vi "4Pi Drift Monitor.vi"() -> ()   [LabVIEW 2021]
uses:
  <vilib>/vision/Image Controls.llb/IMAQ Image.ctl
  4Pi Drift Monitor Controls/4Pi Drift Monitor - Notifier Type.ctl
  4Pi Drift Monitor Controls/4Pi Drift Monitor - Actions.ctl
  Hardware Configuration/Hardware Configuration Controls/Device Type.ctl
  Hardware Configuration/Hardware Configuration Controls/Device Function.ctl
panel:
  in  "CCD Offset":dbl=100.0
  in  "Offset Position Scale":dbl=2.0
  out "ROI Stack":u16[][][](array[numeric])
  out "Y (nm)":cluster{dbl, dbl, dbl, dbl}(graph)
  in  "Quit":bool
  out "Init X pos (px)":dbl[](array[numeric])
  out "Init Y pos (px)":dbl[](array[numeric])
  out "Y pos (px)":dbl[](array[numeric])
  out "X pos (px)":dbl[](array[numeric])
  in  "Frame Accumulation":i32
  in  "ROI Size":i32=7
  in  "Camera Px. Size (nm)":dbl=0.1
  in  "qd4":bool=TRUE
  in  "qd3":bool=TRUE
  in  "qd2":bool=TRUE
  in  "qd1":bool=TRUE
  out "X (nm)":cluster{dbl, dbl, dbl, dbl}(graph)
  in  "Start Monitor":bool
  # "Quadrant"
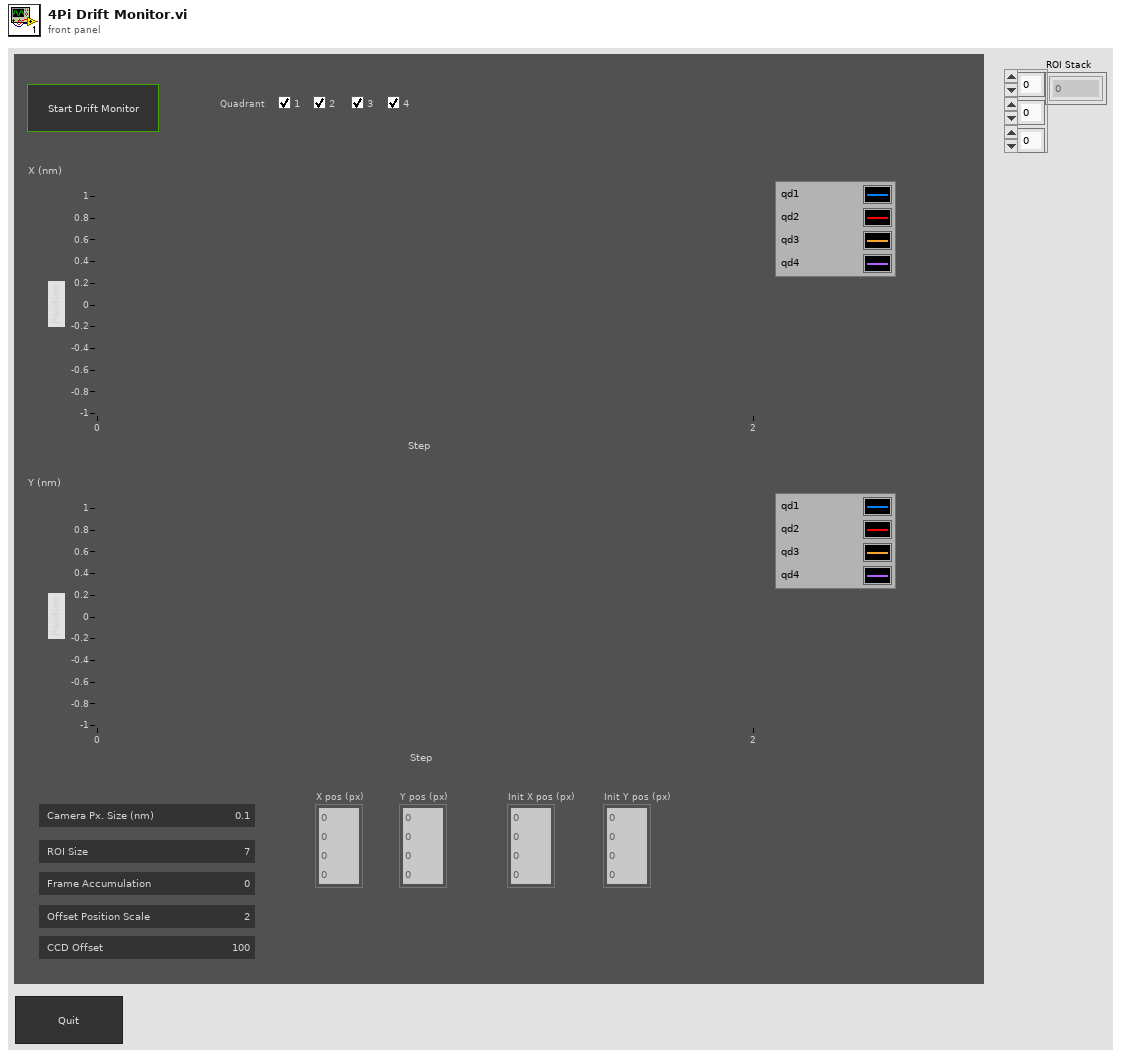
[diagram p1: front panel]
types:
  T1 = typedef "4Pi Drift Monitor - Actions.ctl" = enum16{"Idle", "Start Monitor", "Get Initial XY Pos", "Get Initial Image", "Get Image", "Get XY Position", "Update Plots", "Exit Loop", "Abort", "Quit"}
  T2 = typedef "4Pi Drift Monitor - Notifier Type.ctl" = cluster{"Action":T1, "Frame Accums.":u16, "Camera Px. Size (nm)":dbl, "QD On/Off":bool[], "Image Ref":T3[], "ROI Size":i32, "Frame Accumulation":u16, "ROI Stack":u16[][][], "Running?":bool}
  T3 = typedef "IMAQ Image.ctl" = refnum<image>
  T4 = typedef "Device Function.ctl" = enum16{"Primary", "Secondary", "Overview", "Wide Field Drift Correction", "642 nm Excitation", "560 nm Excitation", "940 nm Excitation", "546 nm Excitation", "488 nm Excitation", "405 nm Excitation", "Objective Drift Correction", "4Pi Focus Lock", "4Pi Objective Lock", "Objective XY", "Objective Z", "Sample XY", "Sample Coarse Z", "Sample Z", "4Pi Lower", "4Pi Upper", "Em Small", "Em Large", "Ex Small", "Ex Large", "Mojo", "Adj Cavity", "Line Scanning", "Alert"}
  T5 = typedef "Device Type.ctl" = enum16{"AOTF", "Camera", "Deformable Mirror", "Laser", "Flip Mirror", "Shutter", "Stage", "Waveform", "FPGA", "Email"}
  T6 = typedef "4Pi OBJ Lock-2D Gaussian - Best Fit Parameters.ctl" = cluster{"Amplitude":dbl, "X Position":dbl, "Y Position":dbl, "X Width":dbl, "Y Width":dbl, "Offset":dbl}
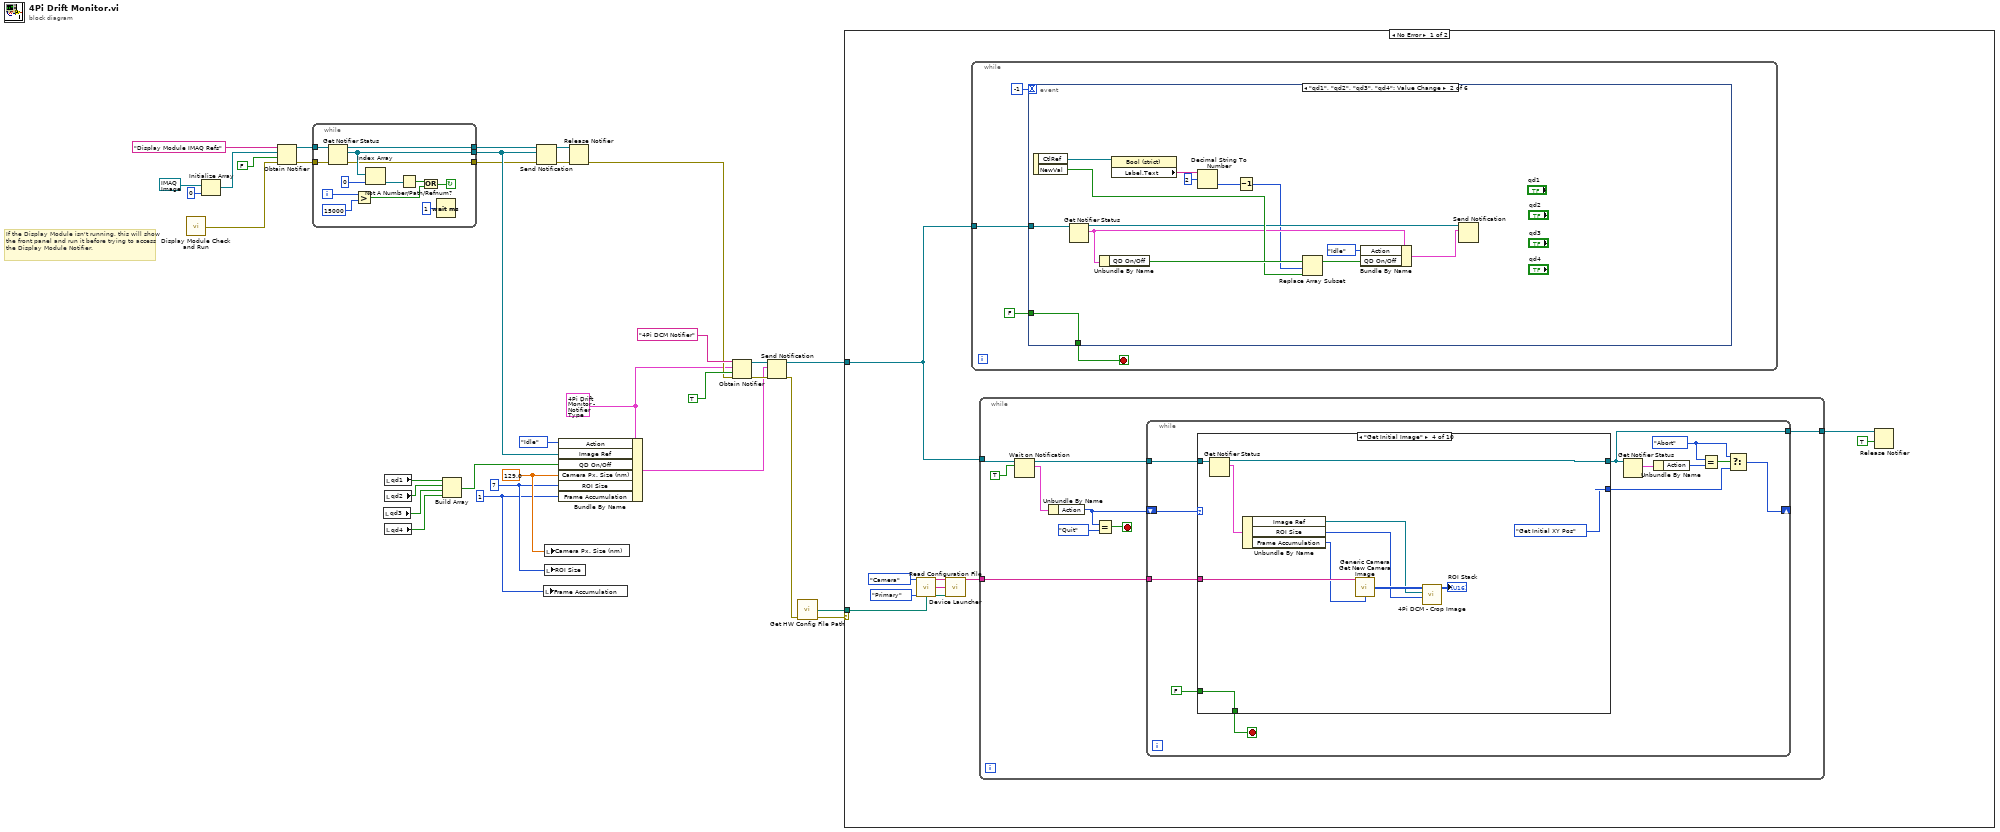
[diagram p0: block diagram]
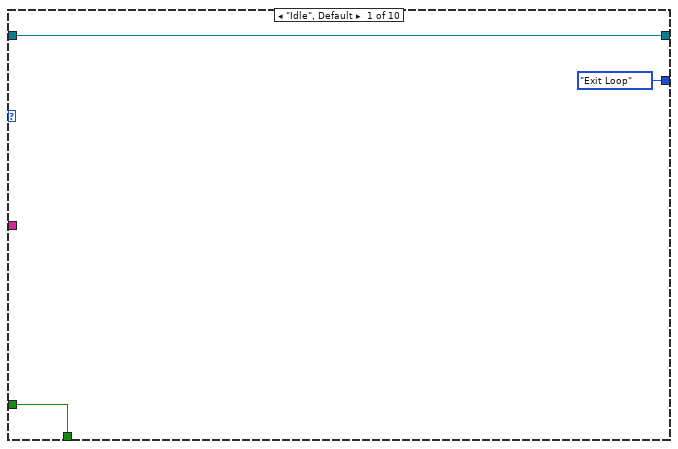
[diagram p2: hidden frame]
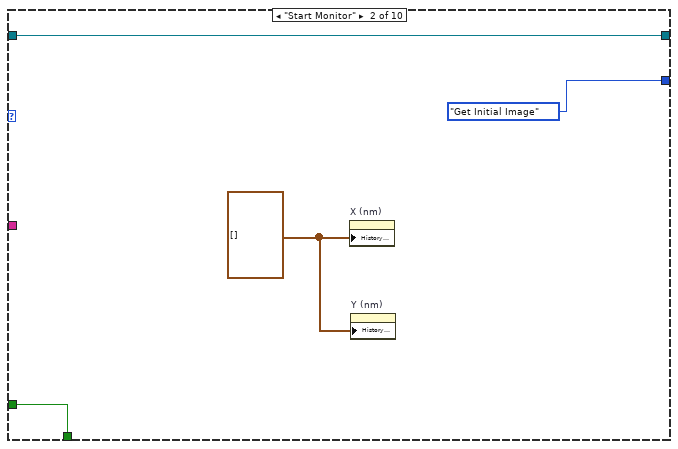
[diagram p3: hidden frame]
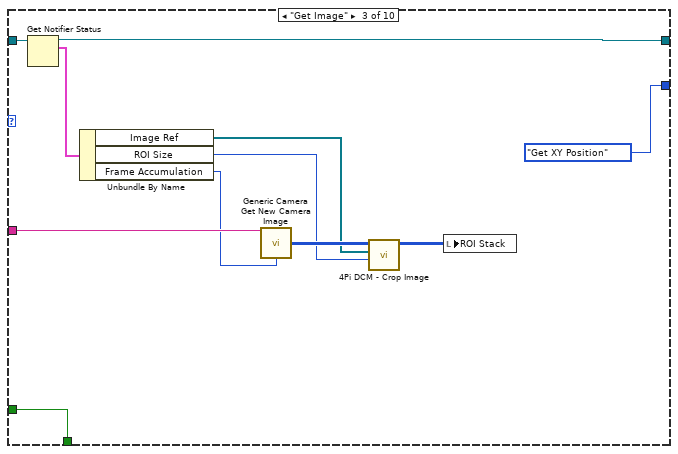
[diagram p4: hidden frame]
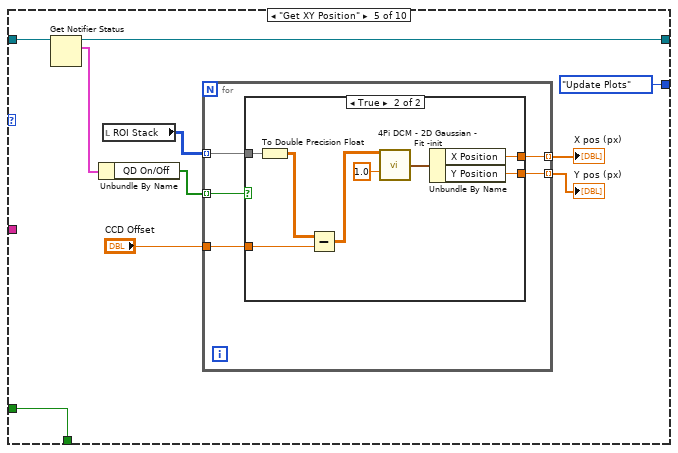
[diagram p5: hidden frame]
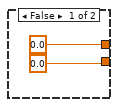
[diagram p6: hidden frame]
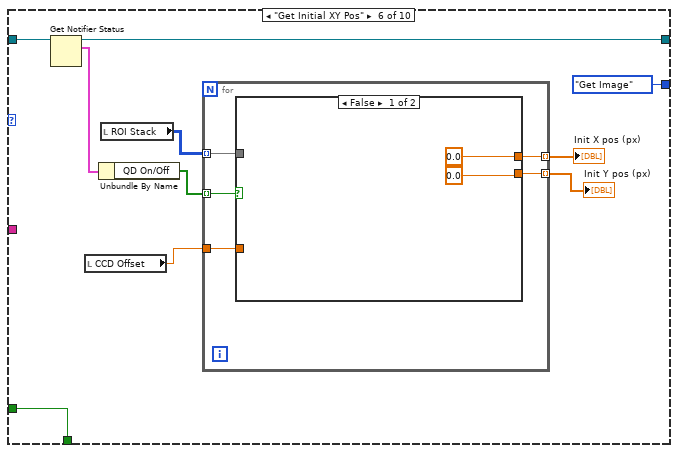
[diagram p7: hidden frame]
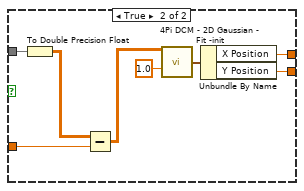
[diagram p8: hidden frame]
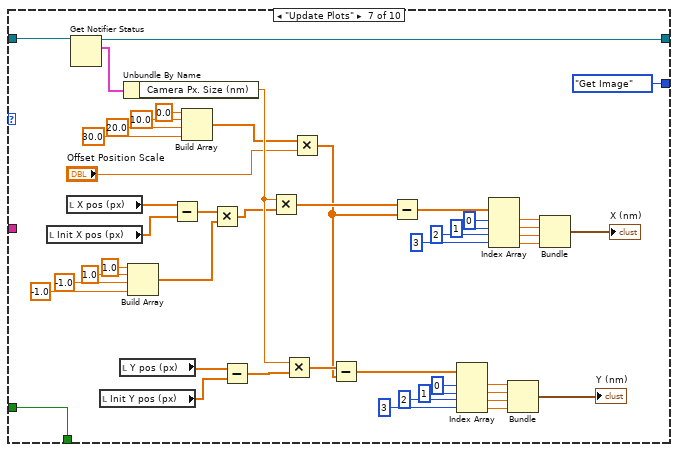
[diagram p9: hidden frame]
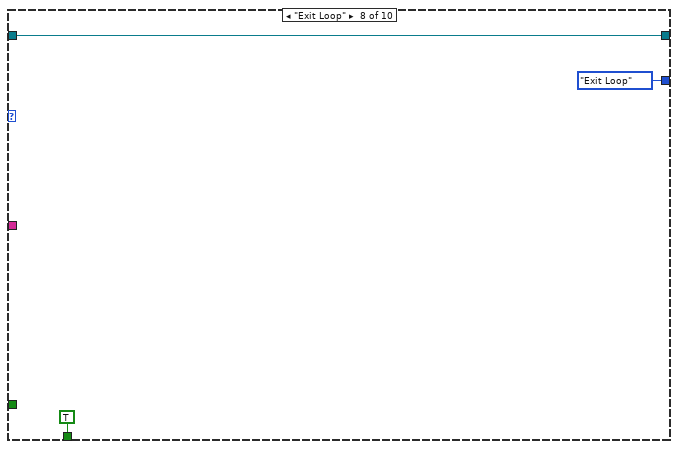
[diagram p10: hidden frame]
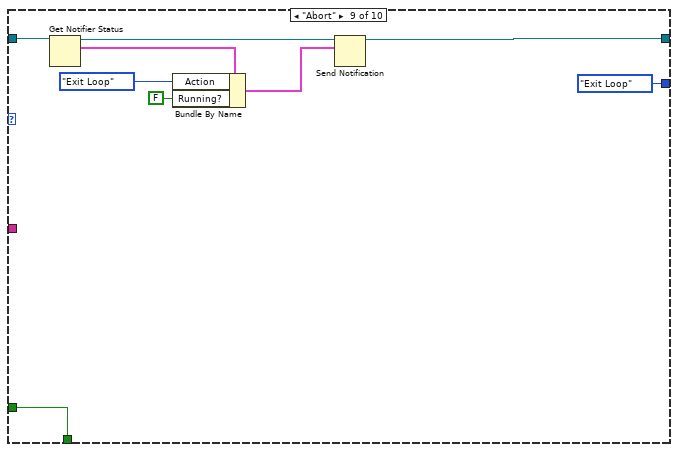
[diagram p11: hidden frame]
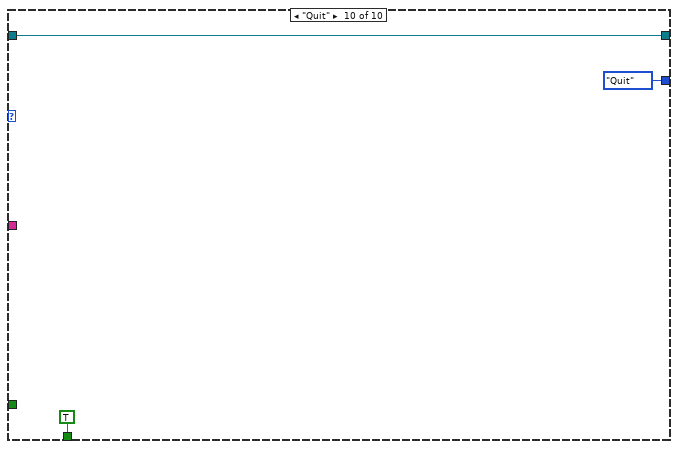
[diagram p12: hidden frame]
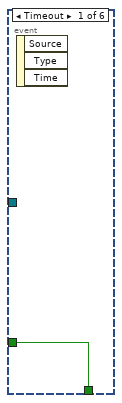
[diagram p13: hidden frame]
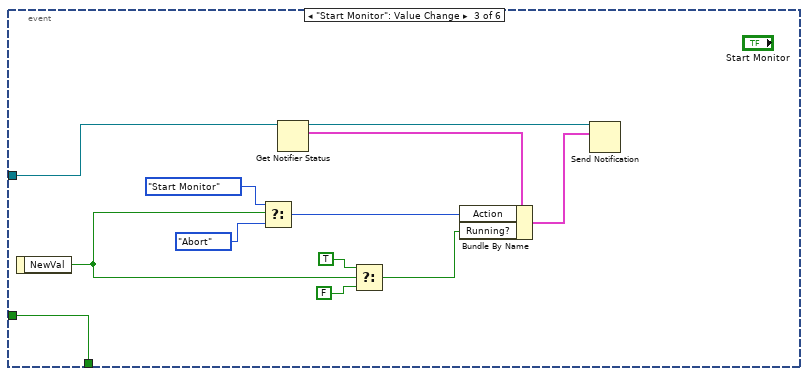
[diagram p14: hidden frame]
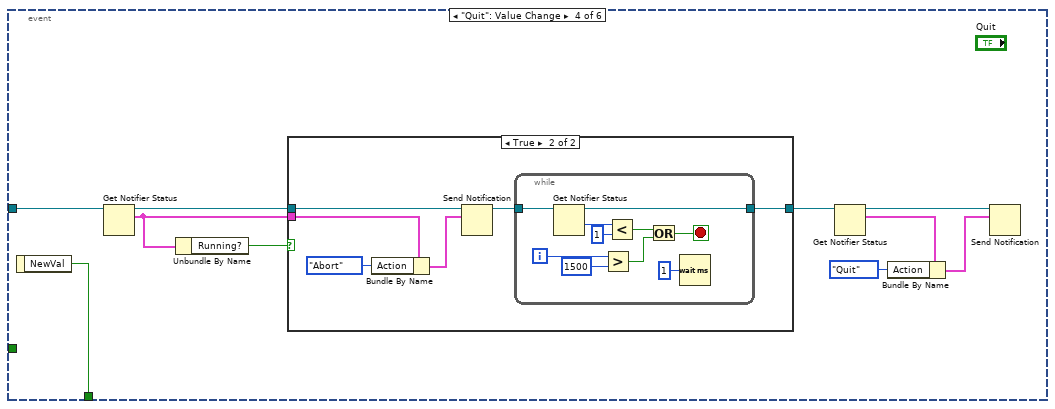
[diagram p15: hidden frame]
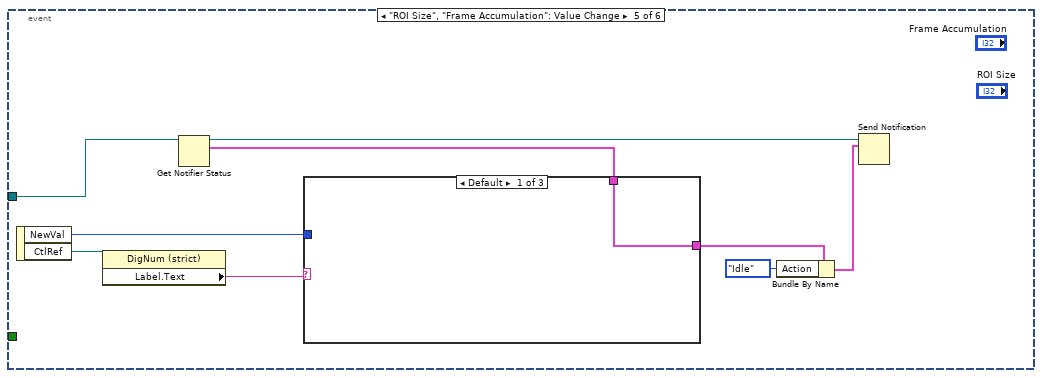
[diagram p17: hidden frame]
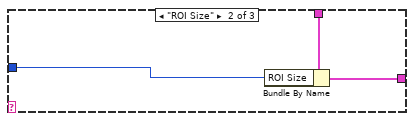
[diagram p18: hidden frame]
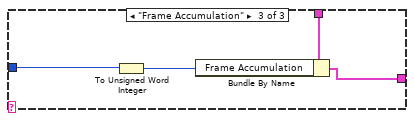
[diagram p19: hidden frame]
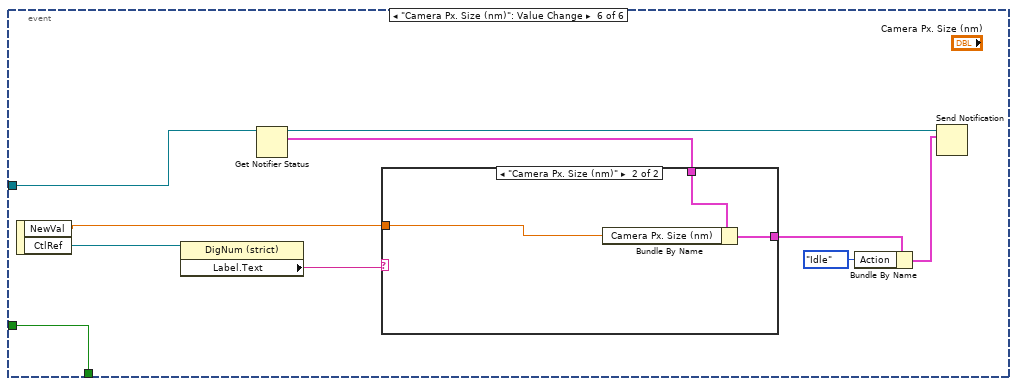
[diagram p20: hidden frame]
diagram:
  w2 = u16 1 ("Frame Accumulation")
  w3 = 7 ("ROI Size")
  w4 = 129.0 ("Camera Px. Size (nm)")
  w1 = T2 {"Action"=enum."Start Monitor", "Frame Accums."=0, "Camera Px. Size (nm)"=0.1, "QD On/Off"=[], "Image Ref"=[], "ROI Size"=0, "Frame Accumulation"=0, "ROI Stack"=[], "Running?"=FALSE} ("4Pi Drift Monitor Notifier Type")
  # "If the Display Module isn't running, this will show the front panel and run it before trying to access the Display Module Notifier."
  n1 = call "Display Module Check and Run.vi"() -> ("Error"=w29:errorcluster)  [unwired: 15 in]
  n2 = Initialize Array(T3 refnum ("New Image"), 0 ("dimension size")) -> (w26:T3[])
  n3 = Obtain Notifier(name (unnamed)="Display Module IMAQ Refs", notification data type=w26, create if not found? (T)=FALSE, error in (no error)=w29) -> (notifier out=w28:refnum<notifier>, error out=w27:errorcluster)  [unwired: 1 out]
  n4 = while {
    tunnel: w28 -> [w46]
    tunnel: w27 -> [w45]
    tunnel: [w44] -> w8
    tunnel: [w43] -> w7
    tunnel: [w39] -> w6
    i -> [w38]
    stop <- w35 continue-if-true
    n5 = Get Notifier Status(notifier=w46, error in (no error)=w45) -> (notifier out=w44:refnum<notifier>, current notification=w43:T3[], error out=w39:errorcluster)  [unwired: 2 out]
    n6 = Greater?(x=w38, y=15000) -> (0:w34:bool)
    n7 = Index Array(array=w43, index=0) -> (element=w41:T3)
    n8 = Not A Number/Path/Refnum?(number/path/refnum=w41) -> (NaN/Path/Refnum?=w36:bool)
    n9 = Or(x=w36, y=w34) -> (x .or. y?=w35:bool)
    n10 = Wait (ms)(milliseconds to wait=u32 1) -> ()  [unwired: 1 out]
  }
  n11 = local read "qd3"() -> (w13:bool)
  n12 = local read "qd1"() -> (w15:bool)
  n13 = local read "qd2"() -> (w14:bool)
  n14 = local read "qd4"() -> (w12:bool)
  n15 = Build Array(w15, w14, w13, w12) -> (w11:bool[])
  n16 = Send Notification(notification=w7, notifier=w8, error in (no error)=w6) -> (notifier out=w9:refnum<notifier>, error out=w10:errorcluster)
  n17 = local write "Frame Accumulation"(w2) -> ()
  n18 = local write "Camera Px. Size (nm)"(w4) -> ()
  n19 = local write "ROI Size"(w3) -> ()
  n20 = Bundle By Name(cluster=w1, "Action"=4Pi_Drift_Monitor_-_Actions."Idle", "Image Ref"=w7, "QD On/Off"=w11, "Camera Px. Size (nm)"=w4, "ROI Size"=w3, "Frame Accumulation"=w2) -> (w17:T2)
  n21 = Release Notifier(notifier=w9, error in (no error)=w10) -> (error out=w5:errorcluster)  [unwired: 1 in, 2 out]
  n22 = Obtain Notifier(name (unnamed)="4Pi DCM Notifier", notification data type=w1, create if not found? (T)=TRUE, error in (no error)=w5) -> (notifier out=w24:refnum<notifier>, error out=w22:errorcluster)  [unwired: 1 out]
  n23 = Send Notification(notification=w17, notifier=w24, error in (no error)=w22) -> (notifier out=w16:refnum<notifier>, error out=w21:errorcluster)
  n24 = call "Get HW Config File Path.vi"("Error"=w21) -> ("File Path"=w19:path, "Error"=w20:errorcluster)  [unwired: 13 in]
  n25 = case shown="No Error" w20 {
    tunnel: w19 -> [w53 _]
    tunnel: w16 -> [w49 _]
    frame No Error {
      n26 = call "Read Configuration File.vi"("Device Type"=Device_Type."Camera", "Device Function"=Device_Function."Primary", "Config File Path"=w53) -> ("Unique Notifier Name"=w54:string, "Device Ports/IDs/Channels"=w56:string[], "Device Engine Path"=w55:path)  [unwired: 9 in, 1 out]
      n27 = call "Device Launcher.vi"("Notifier Name"=w54, "Device Ports/IDs/Channels"=w56, "Device Engine Path"=w55) -> ("Notifier Name"=w50:string)  [unwired: 11 in, 1 out]
      n28 = while {
        tunnel: w49 -> [w222]
        stop <- w221 stop-if-true
        n29 = event shown="[1] \"qd1\", \"qd2\", \"qd3\", \"qd4\": Value Change" {
          selector: _ -> [_ _ _ _ _ _]
          dyn-events: _ -> [_ _ _ _ _ _]
          timeout: -1 -> [_ _ _ _ _ _]
          tunnel: w222 -> [_ w236 w240 w251 w283 w294]
          tunnel: [w223 w226 w243 w259 _ w303] -> w221
          tunnel: FALSE -> [w223 w226 w243 _ _ w303]
          event Timeout {
            n30 = event-data() -> ()  [unwired: 1 in, 3 out]
          }
          event "qd1", "qd2", "qd3", "qd4": Value Change {
            n31 = event-data() -> ("CtlRef"=w237:refnum<vi>, "NewVal"=w232:bool)  [unwired: 1 in]
            n32 = Get Notifier Status(notifier=w236) -> (notifier out=w228:refnum<notifier>, current notification=w231:T2)  [unwired: 1 in, 3 out]
            n33 = Unbundle By Name(w231) -> ("QD On/Off"=w235:bool[])
            n34 = property class="Bool (strict)"(reference=w237) -> ("Label.Text"=w234:string)  [unwired: 1 in, 2 out]
            n35 = Decimal String To Number(string=w234, offset=2 ("offset (0)")) -> (number=w225:i32)  [unwired: 1 in, 1 out]
            n36 = Decrement(x=w225) -> (x-1=w224:i32)
            n37 = Replace Array Subset(array=w235, new element=w232, index=w224) -> (w230:bool[])
            n38 = Bundle By Name(cluster=w231, "Action"=4Pi_Drift_Monitor_-_Actions."Idle", "QD On/Off"=w230) -> (w229:T2)
            n39 = Send Notification(notification=w229, notifier=w228) -> ()  [unwired: 1 in, 2 out]
          }
          event "Start Monitor": Value Change {
            n40 = event-data() -> ("NewVal"=w239:bool)  [unwired: 1 in]
            n41 = Select(t=4Pi_Drift_Monitor_-_Actions."Start Monitor" ("Action"), s=w239, f=4Pi_Drift_Monitor_-_Actions."Abort") -> (s? t:f=w246:T1)
            n42 = Get Notifier Status(notifier=w240) -> (notifier out=w244:refnum<notifier>, current notification=w249:T2)  [unwired: 1 in, 3 out]
            n43 = Select(t=TRUE ("Running?"), s=w239, f=FALSE) -> (s? t:f=w238:bool)
            n44 = Bundle By Name(cluster=w249, "Action"=w246, "Running?"=w238) -> (w245:T2)
            n45 = Send Notification(notification=w245, notifier=w244) -> ()  [unwired: 1 in, 2 out]
          }
          event "Quit": Value Change {
            n46 = event-data() -> ("NewVal"=w259:bool)  [unwired: 1 in]
            n47 = Get Notifier Status(notifier=w251) -> (notifier out=w254:refnum<notifier>, current notification=w252:T2)  [unwired: 1 in, 3 out]
            n48 = Unbundle By Name(w252) -> ("Running?"=w255:bool)
            n49 = case shown="True" w255 {
              tunnel: w254 -> [w260 w265]
              tunnel: [w260 w262] -> w253
              tunnel: w252 -> [_ w266]
              frame False {
              }
              frame True {
                n50 = Bundle By Name(cluster=w266, "Action"=4Pi_Drift_Monitor_-_Actions."Abort") -> (w264:T2)
                n51 = Send Notification(notification=w264, notifier=w265) -> (notifier out=w263:refnum<notifier>)  [unwired: 1 in, 1 out]
                n52 = while {
                  tunnel: w263 -> [w276]
                  tunnel: [w271] -> w262
                  i -> [w270]
                  stop <- w272 stop-if-true
                  n53 = Get Notifier Status(notifier=w276) -> (notifier out=w271:refnum<notifier>, # waiting=w275:i32)  [unwired: 1 in, 3 out]
                  n54 = Greater?(x=w270, y=1500) -> (0:w268:bool)
                  n55 = Less?(x=w275, y=1) -> (x < y?=w273:bool)
                  n56 = Or(x=w273, y=w268) -> (x .or. y?=w272:bool)
                  n57 = Wait (ms)(milliseconds to wait=u32 1) -> ()  [unwired: 1 out]
                }
              }
            }
            n58 = Get Notifier Status(notifier=w253) -> (notifier out=w257:refnum<notifier>, current notification=w258:T2)  [unwired: 1 in, 3 out]
            n59 = Bundle By Name(cluster=w258, "Action"=4Pi_Drift_Monitor_-_Actions."Quit") -> (w256:T2)
            n60 = Send Notification(notification=w256, notifier=w257) -> ()  [unwired: 1 in, 2 out]
          }
          event "ROI Size", "Frame Accumulation": Value Change {
            n61 = event-data() -> ("NewVal"=w281:i32, "CtlRef"=w285:refnum<vi>)  [unwired: 1 in]
            n62 = property class="DigNum (strict)"(reference=w285) -> ("Label.Text"=w284:string)  [unwired: 1 in, 2 out]
            n63 = Get Notifier Status(notifier=w283) -> (notifier out=w280:refnum<notifier>, current notification=w282:T2)  [unwired: 1 in, 3 out]
            n64 = case shown="Default" w284 {
              tunnel: w282 -> [w286 w289 w293]
              tunnel: w281 -> [_ w288 w291]
              tunnel: [w286 w287 w292] -> w279
              frame Default {
              }
              frame "ROI Size" {
                n65 = Bundle By Name(cluster=w289, "ROI Size"=w288) -> (w287:T2)
              }
              frame "Frame Accumulation" {
                n66 = To Unsigned Word Integer(number=w291) -> (unsigned 16bit integer=w290:u16)
                n67 = Bundle By Name(cluster=w293, "Frame Accumulation"=w290) -> (w292:T2)
              }
            }
            n68 = Bundle By Name(cluster=w279, "Action"=4Pi_Drift_Monitor_-_Actions."Idle") -> (w277:T2)
            n69 = Send Notification(notification=w277, notifier=w280) -> ()  [unwired: 1 in, 2 out]
          }
          event "Camera Px. Size (nm)": Value Change {
            n70 = event-data() -> ("NewVal"=w295:dbl, "CtlRef"=w296:refnum<vi>)  [unwired: 1 in]
            n71 = property class="DigNum (strict)"(reference=w296) -> ("Label.Text"=w302:string)  [unwired: 1 in, 2 out]
            n72 = Get Notifier Status(notifier=w294) -> (notifier out=w300:refnum<notifier>, current notification=w301:T2)  [unwired: 1 in, 3 out]
            n73 = case shown="\"Camera Px. Size (nm)\"" w302 {
              tunnel: w301 -> [w304 w307]
              tunnel: w295 -> [_ w306]
              tunnel: [w304 w305] -> w299
              frame Default {
              }
              frame "Camera Px. Size (nm)" {
                n74 = Bundle By Name(cluster=w307, "Camera Px. Size (nm)"=w306) -> (w305:T2)
              }
            }
            n75 = Bundle By Name(cluster=w299, "Action"=4Pi_Drift_Monitor_-_Actions."Idle") -> (w297:T2)
            n76 = Send Notification(notification=w297, notifier=w300) -> ()  [unwired: 1 in, 2 out]
          }
        }
      }
      n77 = while {
        tunnel: w50 -> [w59]
        tunnel: w49 -> [w63]
        tunnel: [w57] -> w47
        stop <- w61 stop-if-true
        n78 = Wait on Notification(notifier=w63, ignore previous (F)=TRUE) -> (notifier out=w60:refnum<notifier>, notification=w64:T2)  [unwired: 2 in, 2 out]
        n79 = Unbundle By Name(w64) -> ("Action"=w58:T1)
        n80 = Equal?(x=w58, y=4Pi_Drift_Monitor_-_Actions."Quit") -> (x = y?=w61:bool)
        n81 = while {
          tunnel: w60 -> [w77]
          tunnel: w59 -> [w76]
          shift-right: [w70] -> _
          shift-left: w58 -> [w69]
          tunnel: [w66] -> w57
          stop <- w68 stop-if-true
          w72 = 4Pi_Drift_Monitor_-_Actions."Abort" ("x")
          n82 = case shown="\"Get Initial Image\"" w69 {
            tunnel: [w79 w84 w86 w97 w111 w136 w177 w206 w209 w216] -> w66
            tunnel: w77 -> [w79 w84 w95 w106 w116 w141 w203 w206 w215 w216]
            tunnel: w76 -> [_ _ w94 w105 _ _ _ _ _ _]
            tunnel: [4Pi_Drift_Monitor_-_Actions."Exit Loop" ("y") 4Pi_Drift_Monitor_-_Actions."Get Initial Image" ("y") 4Pi_Drift_Monitor_-_Actions."Get XY Position" ("y") 4Pi_Drift_Monitor_-_Actions."Get Initial XY Pos" ("y") 4Pi_Drift_Monitor_-_Actions."Update Plots" ("y") 4Pi_Drift_Monitor_-_Actions."Get Image" ("y") 4Pi_Drift_Monitor_-_Actions."Get Image" ("y") 4Pi_Drift_Monitor_-_Actions."Exit Loop" ("y") 4Pi_Drift_Monitor_-_Actions."Exit Loop" ("y") 4Pi_Drift_Monitor_-_Actions."Quit" ("y")] -> w71
            tunnel: [w78 w81 w87 w98 w110 w135 w176 TRUE w208 TRUE] -> w68
            tunnel: FALSE -> [w78 w81 w87 w98 w110 w135 w176 _ w208 _]
            frame "Idle", Default {
            }
            frame "Start Monitor" {
              w82 = cluster{dbl, dbl, dbl, dbl}[] [] ("History Data")
              n83 = property on="X (nm)" class="WFChart (strict)"("History Data"=w82) -> ()  [unwired: 2 in, 2 out]
              n84 = property on="Y (nm)" class="WFChart (strict)"("History Data"=w82) -> ()  [unwired: 2 in, 2 out]
            }
            frame "Get Image" {
              n85 = Get Notifier Status(notifier=w95) -> (notifier out=w86:refnum<notifier>, current notification=w89:T2)  [unwired: 1 in, 3 out]
              n86 = Unbundle By Name(w89) -> ("Image Ref"=w92:T3[], "ROI Size"=w91:i32, "Frame Accumulation"=w90:u16)
              n87 = call "Generic Camera Get New Camera Image.vi"("Camera Notifier Name"=w94, "Frames"=w90) -> ("Image - U16"=w93:u16[][])  [unwired: 11 in, 2 out]
              n88 = call "4Pi DCM - Crop Image.vi"("ROI Size"=w91, "Image Refs"=w92, "Input Image (U16)"=w93) -> ("Output Image Stack"=w85:u16[][][])  [unwired: 8 in]
              n89 = local write "ROI Stack"(w85) -> ()
            }
            frame "Get Initial Image" {
              n90 = Get Notifier Status(notifier=w106) -> (notifier out=w97:refnum<notifier>, current notification=w100:T2)  [unwired: 1 in, 3 out]
              n91 = Unbundle By Name(w100) -> ("Image Ref"=w103:T3[], "ROI Size"=w102:i32, "Frame Accumulation"=w101:u16)
              n92 = call "Generic Camera Get New Camera Image.vi"("Camera Notifier Name"=w105, "Frames"=w101) -> ("Image - U16"=w104:u16[][])  [unwired: 11 in, 2 out]
              n93 = call "4Pi DCM - Crop Image.vi"("ROI Size"=w102, "Image Refs"=w103, "Input Image (U16)"=w104) -> ("Output Image Stack"=→"ROI Stack":u16[][][])  [unwired: 8 in]
            }
            frame "Get XY Position" {
              n94 = Get Notifier Status(notifier=w116) -> (notifier out=w111:refnum<notifier>, current notification=w115:T2)  [unwired: 1 in, 3 out]
              n95 = Unbundle By Name(w115) -> ("QD On/Off"=w109:bool[])
              n96 = local read "ROI Stack"() -> (w108:u16[][][])
              n97 = for {
                tunnel: w108 -> [w121] mode=indexing
                tunnel: [w120] -> w114 mode=indexing
                tunnel: [w119] -> w113 mode=indexing
                tunnel: w109 -> [w118] mode=indexing
                tunnel: "CCD Offset" -> [w117]
                n98 = case shown="True" w118 {
                  tunnel: w121 -> [_ w131]
                  tunnel: [0.0 ("X Position") w128] -> w120
                  tunnel: [0.0 ("Y Position") w127] -> w119
                  tunnel: w117 -> [_ w125]
                  frame False {
                  }
                  frame True {
                    n99 = To Double Precision Float(number=w131) -> (double precision float=w126:dbl[][])
                    n100 = Subtract(x=w126, y=w125) -> (x-y=w124:dbl[][])
                    n101 = call "4Pi DCM - 2D Gaussian - Fit -init.vi"("Image In (DBL)"=w124, "width"=1.0) -> ("Best Fit Params"=w129:T6)  [unwired: 12 in, 1 out]
                    n102 = Unbundle By Name(w129) -> ("X Position"=w128:dbl, "Y Position"=w127:dbl)
                  }
                }
              }
              "X pos (px)" <- w114
              "Y pos (px)" <- w113
            }
            frame "Get Initial XY Pos" {
              n103 = Get Notifier Status(notifier=w141) -> (notifier out=w136:refnum<notifier>, current notification=w140:T2)  [unwired: 1 in, 3 out]
              n104 = local read "CCD Offset"() -> (w132:dbl)
              n105 = Unbundle By Name(w140) -> ("QD On/Off"=w134:bool[])
              n106 = local read "ROI Stack"() -> (w133:u16[][][])
              n107 = for {
                tunnel: w133 -> [w146] mode=indexing
                tunnel: [w145] -> w139 mode=indexing
                tunnel: [w144] -> w138 mode=indexing
                tunnel: w134 -> [w143] mode=indexing
                tunnel: w132 -> [w142]
                n108 = case shown="False" w143 {
                  tunnel: w146 -> [_ w156]
                  tunnel: [0.0 ("X Position") w153] -> w145
                  tunnel: [0.0 ("Y Position") w152] -> w144
                  tunnel: w142 -> [_ w150]
                  frame False {
                  }
                  frame True {
                    n109 = To Double Precision Float(number=w156) -> (double precision float=w151:dbl[][])
                    n110 = Subtract(x=w151, y=w150) -> (x-y=w149:dbl[][])
                    n111 = call "4Pi DCM - 2D Gaussian - Fit -init.vi"("Image In (DBL)"=w149, "width"=1.0) -> ("Best Fit Params"=w154:T6)  [unwired: 12 in, 1 out]
                    n112 = Unbundle By Name(w154) -> ("X Position"=w153:dbl, "Y Position"=w152:dbl)
                  }
                }
              }
              "Init X pos (px)" <- w139
              "Init Y pos (px)" <- w138
            }
            frame "Update Plots" {
              n113 = local read "Init X pos (px)"() -> (w200:dbl[])
              n114 = local read "X pos (px)"() -> (w201:dbl[])
              n115 = Get Notifier Status(notifier=w203) -> (notifier out=w177:refnum<notifier>, current notification=w202:T2)  [unwired: 1 in, 3 out]
              n116 = local read "Init Y pos (px)"() -> (w197:dbl[])
              n117 = local read "Y pos (px)"() -> (w198:dbl[])
              n118 = Unbundle By Name(w202) -> ("Camera Px. Size (nm)"=w196:dbl)
              n119 = Build Array(1.0 ("element"), 1.0 ("element"), -1.0 ("element"), -1.0 ("element")) -> (w158:dbl[])
              n120 = Subtract(x=w201, y=w200) -> (x-y=w159:dbl[])
              n121 = Build Array(0.0 ("element"), 10.0 ("element"), 20.0 ("element"), 30.0 ("element")) -> (w170:dbl[])
              n122 = Multiply(x=w159, y=w158) -> (x*y=w157:dbl[])
              n123 = Subtract(x=w198, y=w197) -> (x-y=w199:dbl[])
              n124 = Multiply(x=w196, y=w157) -> (x*y=w166:dbl[])
              n125 = Multiply(x=w196, y=w199) -> (x*y=w167:dbl[])
              n126 = Multiply(x=w170, y="Offset Position Scale") -> (x*y=w164:dbl[])
              n127 = Subtract(x=w167, y=w164) -> (x-y=w165:dbl[])
              n128 = Subtract(x=w166, y=w164) -> (x-y=w168:dbl[])
              n129 = Index Array(array=w165, index #1=0 ("index"), index #2=1 ("index"), index #3=2 ("index"), index #4=3 ("index")) -> (element #1=w183:dbl, element #2=w182:dbl, element #3=w181:dbl, element #4=w180:dbl)
              n130 = Index Array(array=w168, index #1=0 ("index"), index #2=1 ("index"), index #3=2 ("index"), index #4=3 ("index")) -> (element #1=w191:dbl, element #2=w190:dbl, element #3=w189:dbl, element #4=w188:dbl)
              n131 = Bundle(w183, w182, w181, w180) -> (→"Y (nm)":cluster{dbl, dbl, dbl, dbl})  [unwired: 1 in]
              n132 = Bundle(w191, w190, w189, w188) -> (→"X (nm)":cluster{dbl, dbl, dbl, dbl})  [unwired: 1 in]
            }
            frame "Exit Loop" {
            }
            frame "Abort" {
              n133 = Get Notifier Status(notifier=w215) -> (notifier out=w214:refnum<notifier>, current notification=w213:T2)  [unwired: 1 in, 3 out]
              n134 = Bundle By Name(cluster=w213, "Action"=4Pi_Drift_Monitor_-_Actions."Exit Loop", "Running?"=FALSE) -> (w212:T2)
              n135 = Send Notification(notification=w212, notifier=w214) -> (notifier out=w209:refnum<notifier>)  [unwired: 1 in, 1 out]
            }
            frame "Quit" {
            }
          }
          n136 = Get Notifier Status(notifier=w66) -> (current notification=w75:T2)  [unwired: 1 in, 4 out]
          n137 = Unbundle By Name(w75) -> ("Action"=w73:T1)
          n138 = Equal?(x=w72, y=w73) -> (x = y?=w74:bool)
          n139 = Select(t=w72, s=w74, f=w71) -> (s? t:f=w70:T1)
        }
      }
      n140 = Release Notifier(notifier=w47, force destroy? (F)=TRUE) -> ()  [unwired: 1 in, 3 out]
    }
    frame Error {
      n141 = One Button Dialog(message="Drift Monitor failed to start.") -> ()  [unwired: 1 in, 1 out]
    }
  }
